vi "Read CSM Log Filter Rules.vi"   [LabVIEW 2017, in "INI-Static-Variable-Support.lvlib"]
uses:
  INI-Static-Variable-Support.lvlib
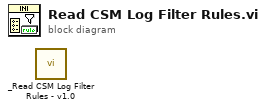
[diagram p0: block diagram]
diagram:
  n1 = call "_Read CSM Log Filter Rules - v1.0.vi"() -> ()  [unwired: 8 in, 4 out]
